vi "HS_Parallel_Port_Client.vi"() -> ()   [LabVIEW 2016]
uses:
  <vilib>/NI/STM/TCP/TCP Read Options.ctl
  <vilib>/NI/STM/TCP/Read Meta Data (TCP Ref).vi
  <vilib>/NI/STM/TCP/Read Meta Data (TCP Clst).vi
  <vilib>/NI/STM/TCP/Read Message (TCP).vi
  <vilib>/NI/STM/TCP/Write Message (TCP).vi
  <vilib>/NI/STM/NI STM.lvlib
panel:
  in  "StepSize":u16=1
  in  "CompArray":u16[](array[numeric])=[0, 1, 2, 3, 4, 5, 6, 7, 8, 9, 10, 11, 12, 13, 14, 15, 16, 17, 18, 19, 20, 21, 22, 23, 24, 25, 26, 27, 28, 29, 30, 31, 32, 33, 34, 35, 36, 37, 38, 39, 40, 41, 42, 43, 44, 45, 46, 47, 48, 49, 50, 51, 52, 53, 54, 55, 56, 57, 58, 59, 60, 61, 62, 63]
  out "Numeric":i32
  out "error":bool
  in  "Check":bool
  in  "file Path":path=path "C:/Users/Erwin/Desktop/refactoring_after_dbg_bus_done"
  in  "Save Button":bool
  in  "StartAcquisition":bool
  out "Actual Depth":u32
  out "Data":u32[](array[numeric]) format="%x"
  out "error out":errorcluster
  in  "Timeout (ms)":i32=5000
  in  "#Samples":u32
  in  "Exit":bool
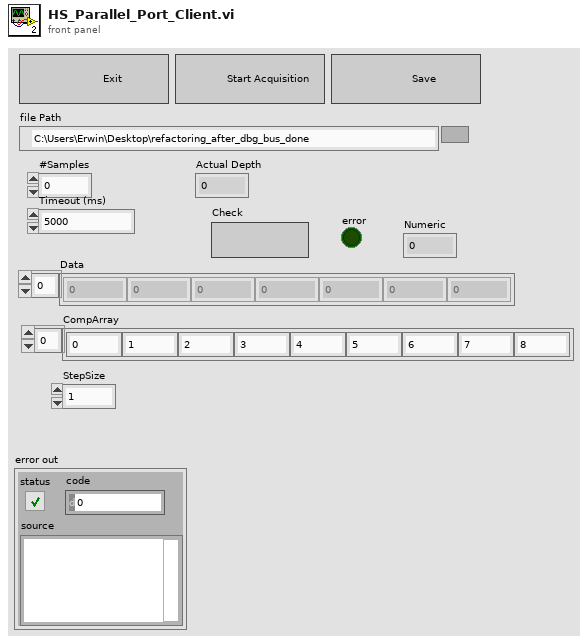
[diagram p1: front panel]
types:
  T1 = typedef "NI STM.lvlib/TCP Read Options.ctl" = cluster{"ignore timeout error":bool, "timeout ms (1000)":i32}
  T2 = enum16{"Read", "Delete", "SetElement", "GetElement", "GetFPelements"}
  T3 = typedef "NI STM.lvlib/MetaDataElement.ctl" = string
  T4 = typedef "NI STM.lvlib/TCP Connection Info.ctl" = cluster{"connection ID":refnum<k5>, "meta data":T3[]}
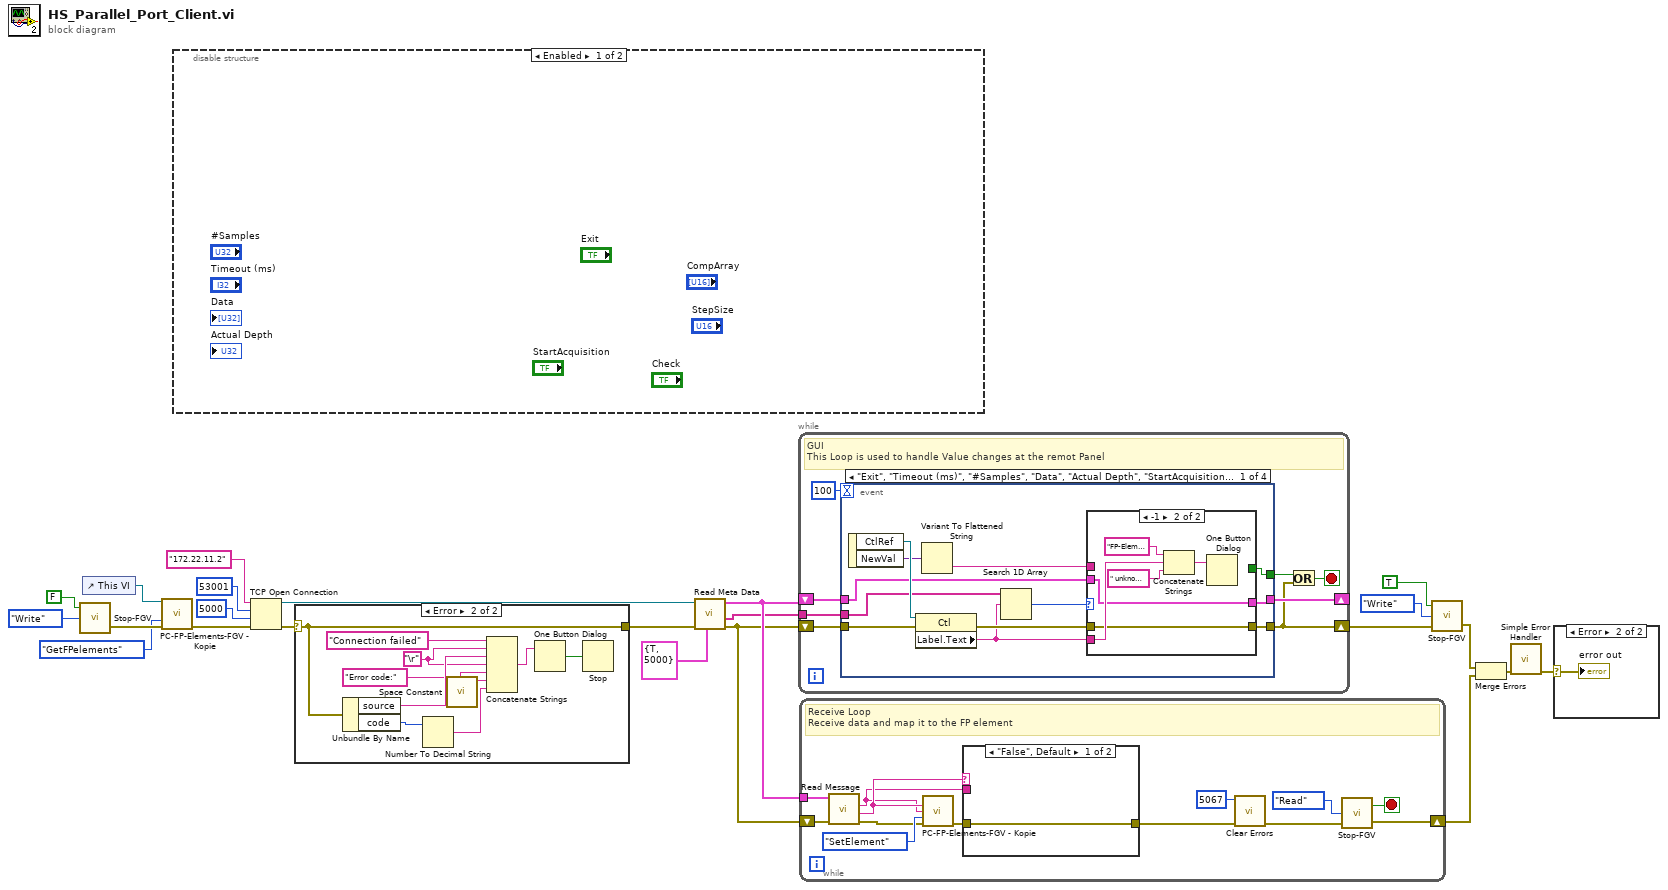
[diagram p0: block diagram]
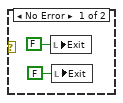
[diagram p3: hidden frame]
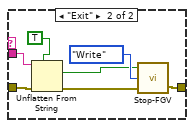
[diagram p4: hidden frame]
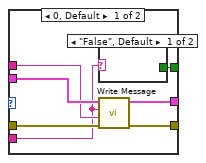
[diagram p5: hidden frame]
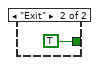
[diagram p6: hidden frame]
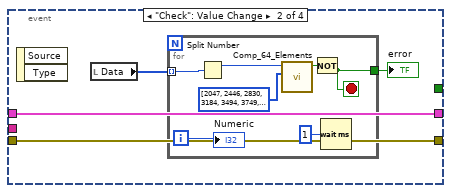
[diagram p7: hidden frame]
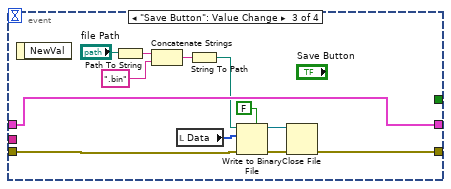
[diagram p8: hidden frame]
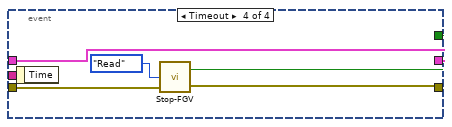
[diagram p9: hidden frame]
diagram:
  n1 = call "Stop-FGV.vi"("Mode"=enum16{"Write", "Read"}."Write", "Stop (in)"=FALSE) -> ("error out"=w3:errorcluster)  [unwired: 1 in, 1 out]
  n2 = control-ref of="This VI"() -> (w4:refnum<vi>)
  n3 = call "PC-FP-Elements-FGV - Kopie.vi"("VI-ref"=w4, "Mode"=T2."GetFPelements", "error in"=w3) -> ("error out"=w1:errorcluster)  [unwired: 8 in, 4 out]
  n4 = disable-structure shown="Enabled" {
    frame Enabled {
    }
    frame Disabled {
    }
  }
  n5 = TCP Open Connection(address="172.22.11.2", remote port or service name=u16 53001, timeout ms (60000)=5000, error in (no error)=w1) -> (connection ID=w20:refnum<k5>, error out=w8:errorcluster)  [unwired: 1 in]
  n6 = case shown="Error" w8 {
    selector: w8 -> [w24 w30]
    tunnel: [w24 w30] -> w7
    frame No Error {
    }
    frame Error {
      w27 = "\r"
      n7 = Unbundle By Name(w30) -> ("source"=w32:string, "code"=w29:i32)
      n8 = Number To Decimal String(number=w29) -> (decimal integer string=w26:string)  [unwired: 1 in]
      n9 = call <vilib>:"Space Constant.vi"() -> ("String"=w25:string)
      n10 = Concatenate Strings("Connection failed", w27, w32, w27, "Error code:", w25, w26) -> (w31:string)
      n11 = One Button Dialog(message=w31) -> (true=w34:bool)  [unwired: 1 in]
      n12 = Stop(stop? (T)=w34) -> ()
    }
  }
  n13 = call-poly <vilib>:"Read Meta Data.vi"("options"=T1 {"ignore timeout error"=TRUE, "timeout ms (1000)"=5000}, "error in"=w7, "connection ID"=w20) -> ("error out"=w10:errorcluster, "meta data"=w5:T3[], "connection info out"=w11:T4)  [unwired: 6 in]
  n14 = while {
    shift-right: [w39] -> _
    shift-left: w11 -> [w40]
    shift-right: [w36] -> w16
    shift-left: w10 -> [w41]
    tunnel: w5 -> [w35]
    stop <- w37 stop-if-true
    # "GUI\nThis Loop is used to handle Value changes at the remot Panel"
    n15 = event shown="[0] \"Exit\", \"Timeout (ms)\", \"#Samples\", \"Data\", \"Actual Depth\", \"StartAcquisition\", \"StepSize\", \"CompArray\": Value Change" {
      selector: _ -> [_ _ _ _]
      dyn-events: _ -> [_ _ _ _]
      timeout: 100 -> [_ _ _ _]
      tunnel: w41 -> [w52 w72 w86 w94]
      tunnel: w40 -> [w50 w71 w91 w96]
      tunnel: [w51 w72 w87 w93] -> w36
      tunnel: [w49 w71 w91 w96] -> w39
      tunnel: [w46 _ _ w92] -> w38
      tunnel: w35 -> [w45 _ _ _]
      event "Exit", "Timeout (ms)", "#Samples", "Data", "Actual Depth", "StartAcquisition", "StepSize", "CompArray": Value Change {
        n16 = event-data() -> ("CtlRef"=w53:refnum<vi>, "NewVal"=w48:variant)  [unwired: 1 in]
        n17 = property class="Ctl"(reference=w53, error in=w52) -> (error out=w54:errorcluster, "Label.Text"=w44:string)  [unwired: 1 out]
        n18 = Variant To Flattened String(Variant=w48) -> (data string=w47:string)  [unwired: 1 out]
        n19 = Search 1D Array(1D array=w45, element=w44) -> (index of element=w43:i32)  [unwired: 1 in]
        n20 = case shown="-1" w43 {
          tunnel: w54 -> [w61 w63]
          tunnel: [w60 w63] -> w51
          tunnel: w50 -> [w59 w64]
          tunnel: [w58 w64] -> w49
          tunnel: w47 -> [w57 _]
          tunnel: [w56 _] -> w46
          tunnel: w44 -> [w55 w67]
          frame 0, Default {
            n21 = case shown="\"False\", Default" w55 {
              tunnel: [_ TRUE] -> w56
              frame "False", Default {
              }
              frame "Exit" {
              }
            }
            n22 = call-poly <vilib>:"Write Message.vi"("error in"=w61, "data"=w57, "name"=w55, "connection info in"=w59) -> ("error out"=w60:errorcluster, "connection info out"=w58:T4)  [unwired: 6 in]
          }
          frame -1 {
            n23 = Concatenate Strings("FP-Element ", w67, " unknown at Target!" ("string")) -> (w65:string)
            n24 = One Button Dialog(message=w65) -> ()  [unwired: 1 in, 1 out]
          }
        }
      }
      event "Check": Value Change {
        n25 = event-data() -> ()  [unwired: 1 in, 2 out]
        n26 = local read "Data"() -> (w70:u32[])
        n27 = for {
          tunnel: w70 -> [w79] mode=indexing
          tunnel: [w75] -> w69
          i -> [w74]
          stop <- w75 stop-if-true
          n28 = Split Number(x=w79) -> (hi(x)=w78:u16)  [unwired: 1 out]
          n29 = call "Comp_64_Elements.vi"("Array"=u16[] [2047, 2446, 2830, 3184, 3494, 3749, 3938, 4055, 4094, 4055, 3938, 3749, 3494, 3184, 2830, 2446, 2047, 1648, 1264, 910, 600, 345, 156, 39, 0, 39, 156, 345, 600, 910, 1264, 1648, 2047, 2446, 2830, 3184, 3494, 3749, 3938, 4055, 4094, 4055, 3938, 3749, 3494, 3184, 2830, 2446, 2047, 1648, 1264, 910, 600, 345, 156, 39, 0, 39, 156, 345, 600, 910, 1264, 1648] ("CompArray"), "CompVal"=w78) -> ("Boolean"=w76:bool)  [unwired: 9 in]
          n30 = Not(x=w76) -> (.not. x?=w75:bool)
          n31 = Wait (ms)(milliseconds to wait=u32 1) -> ()  [unwired: 1 out]
          "Numeric" <- w74
        }
        "error" <- w69
      }
      event "Save Button": Value Change {
        n32 = event-data() -> ()  [unwired: 1 in, 1 out]
        n33 = Path To String(path="file Path") -> (string=w84:string)
        n34 = Concatenate Strings(w84, ".bin" ("name or relative path")) -> (w82:string)
        n35 = local read "Data"() -> (w90:u32[])
        n36 = String To Path(string=w82) -> (path=w81:path)
        n37 = Write to Binary File(file (use dialog)=w81, data=w90, error in=w86, 5:FALSE ("prepend array or string size? (T)")) -> (refnum out=w89:refnum<file>, error out=w88:errorcluster)  [unwired: 2 in, 1 out]
        n38 = Close File(refnum=w89, error in=w88) -> (error out=w87:errorcluster)  [unwired: 1 out]
      }
      event Timeout {
        n39 = event-data() -> ()  [unwired: 1 in, 1 out]
        n40 = call "Stop-FGV.vi"("error in"=w94, "Mode"=enum16{"Write", "Read"}."Read") -> ("error out"=w93:errorcluster, "Stop (out)"=w92:bool)  [unwired: 1 in]
      }
    }
    n41 = Or(x=w38, y=w36) -> (x .or. y?=w37:bool)
  }
  n42 = while {
    tunnel: w11 -> [w109]
    shift-right: [w105] -> w19
    shift-left: w10 -> [w108]
    stop <- w106 stop-if-true
    # "Receive Loop\nReceive data and map it to the FP element"
    n43 = call-poly <vilib>:"Read Message.vi"("error in"=w108, "connection info in"=w109) -> ("error out"=w99:errorcluster, "name"=w102:T3, "data string"=w101:string)  [unwired: 4 in, 3 out]
    n44 = call "PC-FP-Elements-FGV - Kopie.vi"("Name"=w102, "Value in"=w101, "Mode"=T2."SetElement", "error in"=w99) -> ("error out"=w98:errorcluster)  [unwired: 7 in, 4 out]
    n45 = case shown="\"False\", Default" w102 {
      tunnel: [w110 w112] -> w107
      tunnel: w98 -> [w110 w117]
      tunnel: w101 -> [_ w116]
      frame "False", Default {
      }
      frame "Exit" {
        n46 = Unflatten From String(type=TRUE, binary string=w116, error in (no error)=w117) -> (value=w111:bool, error out=w113:errorcluster)  [unwired: 2 in, 1 out]
        n47 = call "Stop-FGV.vi"("error in"=w113, "Mode"=enum16{"Write", "Read"}."Write", "Stop (in)"=w111) -> ("error out"=w112:errorcluster)  [unwired: 1 out]
      }
    }
    n48 = call <vilib>:"Clear Errors.vi"("error in (no error)"=w107, "specific error code to clear (0: all)"=5067) -> ("error out"=w104:errorcluster)  [unwired: 4 in, 1 out]
    n49 = call "Stop-FGV.vi"("error in"=w104, "Mode"=enum16{"Write", "Read"}."Read") -> ("error out"=w105:errorcluster, "Stop (out)"=w106:bool)  [unwired: 1 in]
  }
  n50 = call "Stop-FGV.vi"("error in"=w16, "Mode"=enum16{"Write", "Read"}."Write", "Stop (in)"=TRUE) -> ("error out"=w15:errorcluster)  [unwired: 1 out]
  n51 = Merge Errors(w15, w19) -> (w18:errorcluster)
  n52 = call <vilib>:"Simple Error Handler.vi"("error in (no error)"=w18) -> ("error out"=w9:errorcluster)  [unwired: 4 in, 4 out]
  n53 = case shown="Error" w9 {
    selector: w9 -> [_ w120]
    frame No Error {
      n54 = local write "Exit"(FALSE ("Exit")) -> ()
      n55 = local write "Exit"(FALSE ("Exit")) -> ()
    }
    frame Error {
      "error out" <- w120
    }
  }
